vi "niRFUtil MASMT Resample (constant to constant)_Resample (MultiCh, CSG).vi"(4 "max decimation":i32=1000, 6 "Resample FIR":sgl[](array[numeric]), 7 "reset?":bool, 8 "error in (no error)":errorcluster, 9 "config":T1 {"timing jitter" items=["Interpolation", "Rounding"]}, 10 "anti-aliasing?":bool=TRUE, 11 "X":csg[][](array[numeric])) -> (0 "error out":errorcluster, 2 "t0":sgl, 3 "Y":csg[][](array[numeric]))   [LabVIEW 2015, in "niRFUtil.lvlib"]
uses:
  niRFUtil.lvlib
  Utilities/niRFMASMT_FFT.dll
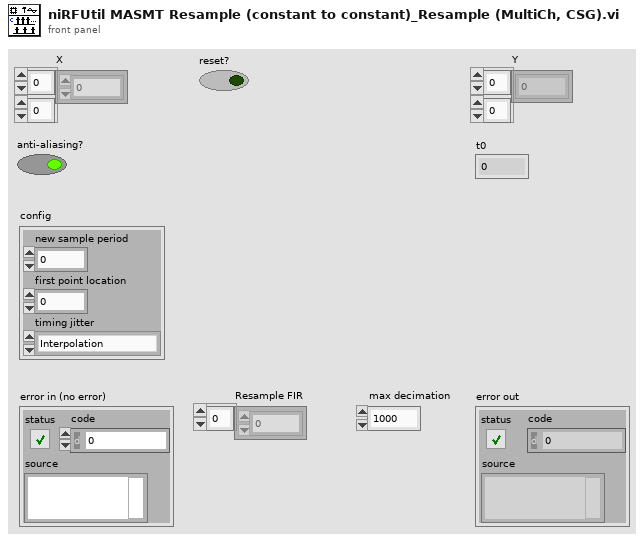
[diagram p1: front panel]
types:
  T1 = cluster{"new sample period":sgl, "first point location":sgl, "timing jitter":i32}
  T2 = cluster{"preConditionLen":i32, "extractFilterLeftLen":i32, "extractFilterRightLen":i32, "extractFilterMethod":i32, "extractFilterScaling":dbl, "samplingPeriod":dbl, "startTime":dbl, "offset":dbl, "index":i32}
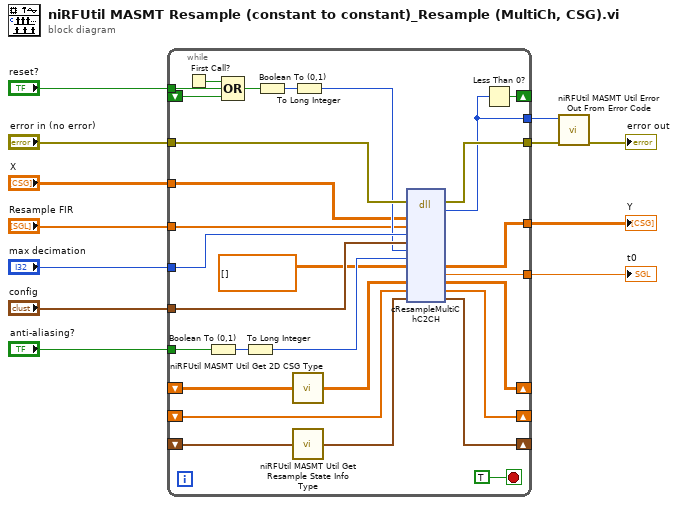
[diagram p0: block diagram]
diagram:
  n1 = while {
    tunnel: "X" -> [w13]
    tunnel: "config" -> [w41]
    tunnel: "error in (no error)" -> [w40]
    tunnel: [w39] -> w1
    tunnel: "anti-aliasing?" -> [w38]
    tunnel: "Resample FIR" -> [w17]
    tunnel: "max decimation" -> [w36]
    tunnel: [w25] -> w12
    tunnel: [w34] -> w11
    tunnel: [w33] -> w2
    tunnel: "reset?" -> [w23]
    shift-right: [w30] -> _
    shift-left: _ -> [w15]
    shift-right: [w31] -> _
    shift-left: _ -> [w27]
    shift-right: [w24] -> _
    shift-left: _ -> [w22]
    shift-right: [w29] -> _
    shift-left: _ -> [w18]
    stop <- TRUE stop-if-true
    n2 = First Call?() -> (First Call?: T/F=w19:bool)
    n3 = Boolean To (0,1)(Boolean=w38) -> (0, 1=w37:i16)
    n4 = Compound Arithmetic op=OR(w19, w23, w22) -> (w20:bool)
    n5 = To Long Integer(number=w37) -> (32bit integer=w35:i32)
    n6 = Boolean To (0,1)(Boolean=w20) -> (0, 1=w21:i16)
    n7 = call "niRFUtil MASMT Util Get 2D CSG Type.vi"("2D CSG Array in"=w15) -> ("2D CSG Array out"=w14:csg[][])
    n8 = call "niRFUtil MASMT Util Get Resample State Info Type.vi"("resample state info in"=w27) -> ("resample state info out"=w26:T2)
    n9 = To Long Integer(number=w21) -> (32bit integer=w32:i32)
    n10 = dll-call lib="C:/Perforce/semoore-sales/Customers/NATI-3813/Noise Floor/LV Filters/ParallelComplexFilterRFUtil/niRFUtil/MASMT/Utilities/niRFMASMT_FFT.*" fn="cResampleMultiChC2CH"(error in=w40, "xH"=w13, "pfilterCoefH"=w17, "pfilterMaxDecimation"=w36, "config"=w41, "reset"=w32, "bandLimit"=w35, "yH"=csg[][] [], "xBufferH"=w14, "extractFilterH"=w18, "state"=w26) -> (error out=w34:errorcluster, "error"=w25:i32, "yH"=w33:csg[][], "t0"=w39:sgl, "xBufferH"=w30:csg[][], "extractFilterH"=w29:sgl[], "state"=w31:T2)  [unwired: 9 in, 1 out]
    n11 = Less Than 0?(x=w25) -> (x < 0?=w24:bool)
  }
  "t0" <- w1
  "Y" <- w2
  n12 = call "niRFUtil MASMT Util Error Out From Error Code.vi"("error in (no error)"=w11, "error code"=w12) -> ("error out"=→"error out":errorcluster)  [unwired: 9 in]
